vi "Stage 4.2 Adding hardware simulation.vi"() -> ()   [LabVIEW 2020]
panel:
  in  "HW type":enum16{"Simulation", "DAQmx", ""}(ring)
  out "Process Error":errorcluster
  out "error out":errorcluster
  out "error out Hardware":errorcluster
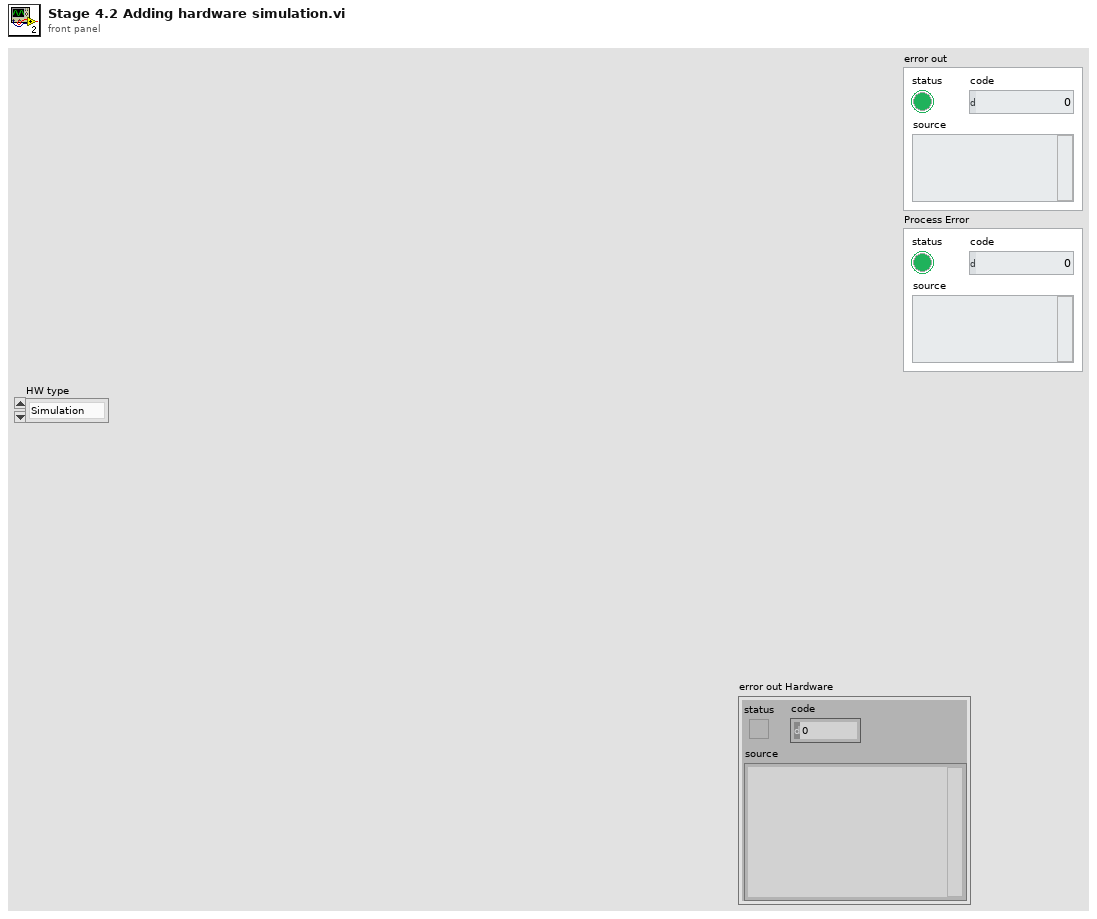
[diagram p1: front panel]
types:
  T1 = typedef "HRM-Stage4-init_cluster.ctl" = cluster{"User Events":T2}
  T2 = typedef "HRM-Stage4-User_events.ctl" = cluster{"Signal to remove":refnum<user-event>, "Sample size":refnum<user-event>, "Filtered wf":refnum<user-event>, "Unfiltered wf":refnum<user-event>, "Raw wf":refnum<user-event>, "Pulse":refnum<user-event>, "Stop":refnum<user-event>, "Feedback":refnum<user-event>, "Run Aqn?":refnum<user-event>}
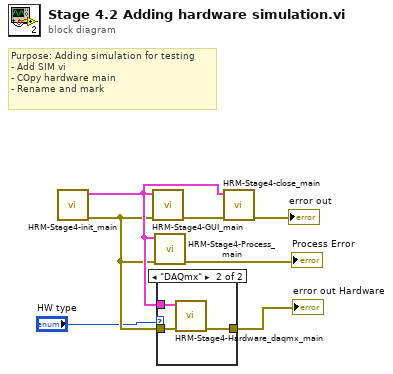
[diagram p0: block diagram]
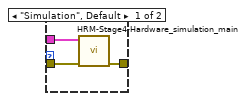
[diagram p2: hidden frame]
diagram:
  # "Purpose: Adding simulation for testing\n- Add SIM vi\n- COpy hardware main\n- Rename and mark"
  n1 = call "HRM-Stage4-init_main.vi"() -> ("error out"=w2:errorcluster, "Init cluster"=w3:T1)  [unwired: 10 in]
  n2 = call "HRM-Stage4-GUI_main.vi"("error in (no error)"=w2, "Init cluster"=w3) -> ("error out"=w4:errorcluster)  [unwired: 9 in]
  n3 = call "HRM-Stage4-Process_main.vi"("error in (no error)"=w2, "Init cluster"=w3) -> ("error out"=→"Process Error":errorcluster)  [unwired: 9 in]
  n4 = case shown="\"DAQmx\"" "HW type" {
    tunnel: [w8 w13] -> w5
    tunnel: w3 -> [w9 w12]
    tunnel: w2 -> [w10 w11]
    frame "Simulation", Default {
      n5 = call "HRM-Stage4-Hardware_simulation_main.vi"("error in (no error)"=w10, "Init cluster"=w9) -> ("error out"=w8:errorcluster)  [unwired: 9 in]
    }
    frame "DAQmx" {
      n6 = call "HRM-Stage4-Hardware_daqmx_main.vi"("error in (no error)"=w11, "Init cluster"=w12) -> ("error out"=w13:errorcluster)  [unwired: 9 in]
    }
  }
  "error out Hardware" <- w5
  n7 = call "HRM-Stage4-close_main.vi"("error in (no error)"=w4, "Init cluster"=w3) -> ("error out"=→"error out":errorcluster)  [unwired: 9 in]
